vi "Performance Formatting Tests.vi"() -> ()   [LabVIEW 2021]
doc: "Measure the duration of <b>Generate Error</b> function with 10, 100 and 1000 input values to be formatted into error description. The resulting durations are returned as an fixed size array (3) where 1st value is for 10 inputs, 2nd for 100 and 3rd for 1000 inputs."
panel:
  out "Duration of formatting 10, 100, 1000 inputs":dbl[](array[numeric])
  in  "error in":errorcluster
  # "Measure the duration of Generate Error function with 10, 100 and 1000 input values to be formatted into error description. The resulting durations are returned as an fixed size array (3) where 1st value is for 10 inputs, 2nd for 100 and 3rd for 1000 inputs."
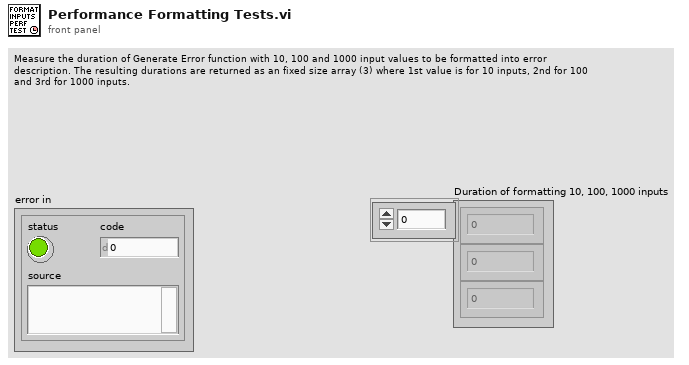
[diagram p1: front panel]
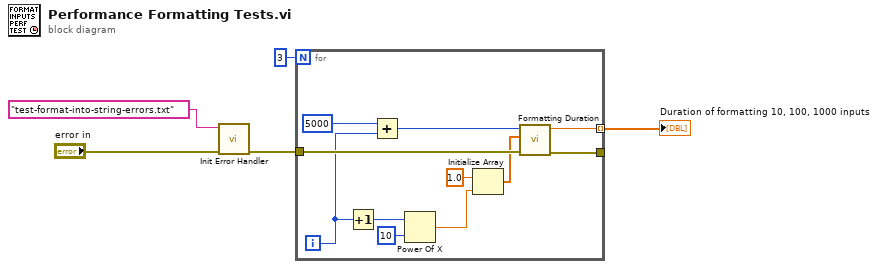
[diagram p0: block diagram]
diagram:
  n1 = call "Init Error Handler.vi"("error in"="error in", "File Prefix Name (Optional)"="test-format-into-string-errors.txt" ("File Name (Optional)")) -> ("error out"=w5:errorcluster)  [unwired: 9 in]
  n2 = for {
    N: 3 -> [_]
    tunnel: w5 -> [w16]
    tunnel: [w13] -> w1 mode=indexing
    tunnel: [w6] -> _
    i -> [w10]
    n3 = Increment(x=w10) -> (x+1=w7:i32)
    n4 = Add(x=5000, y=w10) -> (x+y=w14:i32)
    n5 = Power Of X(1:10 ("x"), 2:w7) -> (0:w8:dbl)
    n6 = Initialize Array(1.0 ("element"), w8) -> (w11:dbl[])
    n7 = call "Formatting Duration.vi"("error in"=w16, "Error Input Values"=w11, "Error Code"=w14) -> ("Generated Error"=w6:errorcluster, "Formatting Generation Duration [ms]"=w13:dbl)  [unwired: 7 in]
  }
  "Duration of formatting 10, 100, 1000 inputs" <- w1
